vi "PH_PILS.set i attribute.vi"(0 "i ref in":refnum<vi>, 2 "i attribute":T1={"Boolean"=[], "GUI Refs Exp. Shutters"={"1"=refnum, "2"=refnum, "3"=refnum, "4"=refnum}, "Tristate2Run GUI Refs"=[], "EO-Likes"=[], "Operation Mode"={"Operation Mode"=enum."unknown", "GUI"={"Ref State"=refnum, "Ref"=refnum}, "Servicemode"={"Tagname"="", "Status"=0}, "Labormode"={"Tagname"="", "Status"=0}, "Searchmode"={"Tagname"="", "Status"=0}, "Shotmode"={"Tagname"="", "Status"=0}}, "Submode"={"Submode"=enum."unknown", "GUI"={"Ref State"=refnum, "Ref"=refnum}, "Submode"={"Tagname"="", "Status"=0}}, "Experiment"={"Experiment"=enum."unknown", "GUI"={"Ref State"=refnum, "Ref"=refnum}, "intern"={"Tagname"="", "Status"=0}, "Exp 4"={"Tagname"="", "Status"=0}, "Exp 3"={"Tagname"="", "Status"=0}, "Exp 2"={"Tagname"="", "Status"=0}, "Exp 1"={"Tagname"="", "Status"=0}}, "TristateNormal"=[], "Door Tags"=[], "GUIlessTags"=[], "Beamline GUI Refs"=[], "Special Boolean"=[], "Laserpower"=[], "Shutter"=[], "Tristate EO Like"=[], "PP"=[], "Switch Knobs"=[], "Latch Knob GUI Refs"=[], "FailureCounter"=0, "Enabled Status"={"Laser"=0, "PreAmp"=0, "MainAmp"=0}, "Mercury"=refnum, "Instance Rods"="N/A", "Logfile"=path "", "Beckhoff-Instance Internal"="", "Beckhoff-Instance External"="", "Enabling Rights"=[]}, 5 "error in (no error)":errorcluster) -> (14 "i ref out":refnum<vi>, 19 "error out":errorcluster)   [LabVIEW 2014, in "PH_PILS.lvlib"]
doc: "Sets the i attribute data of an object.\n\nLicense Agreement for this software:\n\nCopyright (C)\nGesellschaft für Schwerionenforschung, GSI\nPlanckstr. 1\n64291 Darmstadt\nGermany\n\nContact: D.Beck@gsi.de \n\nThis program is free software; you can redistribute it and/or modify it under the terms of the GNU General Public License as published by the Free Software Foundation; either version 2 of the license, or (at your option) any later version.\n\nThis program is distributed in the hope that it will be useful, but WITHOUT ANY WARRANTY; without even the implied warranty of MERCHANTABILITY or FITNESS FOR A PARTICULAR PURPOSE. See the GNU General License for more details (http://www.gnu.org).\n\nGesellschaft für Schwerionenforschung, GSI\nPlanckstr. 1, 64291 Darmstadt, Germany\nFor all questions and ideas contact: M.Richter@gsi.de, H.Brand@gsi.de or D.Beck@gsi.de.\nLast update: 17-JUN-2004"
uses:
  PH_PILS.lvlib
  PH_PILS.i attribute.ctl
  PH_PILS.Operation Mode.ctl
  PH_PILS.Submode.ctl
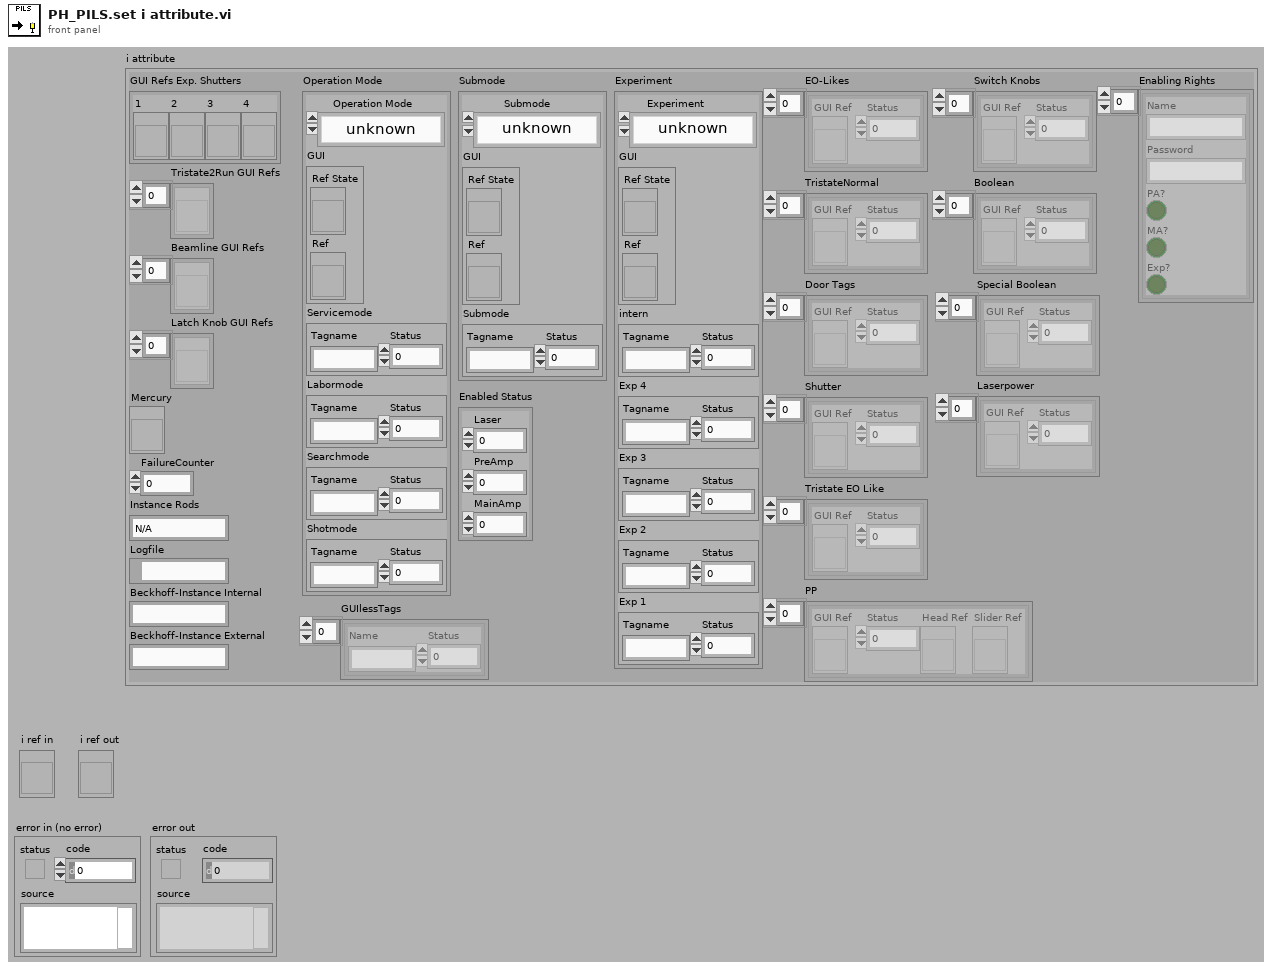
[diagram p1: front panel]
types:
  T1 = typedef "PH_PILS.lvlib/PH_PILS.i attribute.ctl" = cluster{"Boolean":cluster{"GUI Ref":refnum<vi>, "Status":i32}[], "GUI Refs Exp. Shutters":cluster{"1":refnum<vi>, "2":refnum<vi>, "3":refnum<vi>, "4":refnum<vi>}, "Tristate2Run GUI Refs":refnum<vi>[], "EO-Likes":cluster{"GUI Ref":refnum<vi>, "Status":i32}[], "Operation Mode":cluster{"Operation Mode":T2, "GUI":cluster{"Ref State":refnum<vi>, "Ref":refnum<vi>}, "Servicemode":cluster{"Tagname":string, "Status":i32}, "Labormode":cluster{"Tagname":string, "Status":i32}, "Searchmode":cluster{"Tagname":string, "Status":i32}, "Shotmode":cluster{"Tagname":string, "Status":i32}}, "Submode":cluster{"Submode":T3, "GUI":cluster{"Ref State":refnum<vi>, "Ref":refnum<vi>}, "Submode":cluster{"Tagname":string, "Status":i32}}, "Experiment":cluster{"Experiment":enum16{"unknown", "intern", "4 (Z6)", "3", "2", "1"}, "GUI":cluster{"Ref State":refnum<vi>, "Ref":refnum<vi>}, "intern":cluster{"Tagname":string, "Status":i32}, "Exp 4":cluster{"Tagname":string, "Status":i32}, "Exp 3":cluster{"Tagname":string, "Status":i32}, "Exp 2":cluster{"Tagname":string, "Status":i32}, "Exp 1":cluster{"Tagname":string, "Status":i32}}, "TristateNormal":cluster{"GUI Ref":refnum<vi>, "Status":i32}[], "Door Tags":cluster{"GUI Ref":refnum<vi>, "Status":i32}[], "GUIlessTags":cluster{"Name":string, "Status":i32}[], "Beamline GUI Refs":refnum<vi>[], "Special Boolean":cluster{"GUI Ref":refnum<vi>, "Status":i32}[], "Laserpower":cluster{"GUI Ref":refnum<vi>, "Status":i32}[], "Shutter":cluster{"GUI Ref":refnum<vi>, "Status":i32}[], "Tristate EO Like":cluster{"GUI Ref":refnum<vi>, "Status":i32}[], "PP":cluster{"GUI Ref":refnum<vi>, "Status":i32, "Head Ref":refnum<vi>, "Slider Ref":refnum<vi>}[], "Switch Knobs":cluster{"GUI Ref":refnum<vi>, "Status":i32}[], "Latch Knob GUI Refs":refnum<vi>[], "FailureCounter":i32, "Enabled Status":cluster{"Laser":i32, "PreAmp":i32, "MainAmp":i32}, "Mercury":refnum<vi>, "Instance Rods":string, "Logfile":path, "Beckhoff-Instance Internal":string, "Beckhoff-Instance External":string, "Enabling Rights":cluster{"Name":string, "Password":string, "PA?":bool, "MA?":bool, "Exp?":bool}[]}
  T2 = typedef "PH_PILS.lvlib/PH_PILS.Operation Mode.ctl" = enum16{"unknown", "Service", "Labor", "Search", "Shot"}
  T3 = typedef "PH_PILS.lvlib/PH_PILS.Submode.ctl" = enum16{"unknown", "HV-Normal", "HV-Test"}
  T4 = enum16{"SetAttribute", "GetAttribute", "CreateAttribute", "DestroyAttribute", "DestroyAllAtributes"}
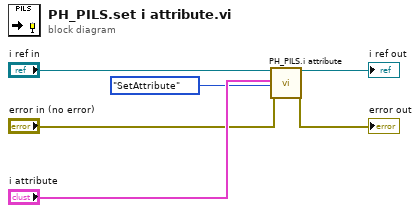
[diagram p0: block diagram]
diagram:
  n1 = call "PH_PILS.i attribute.vi"("VI Refnum"="i ref in", "CLASS.i attribute"="i attribute", "Action"=T4."SetAttribute", "error in (no error)"="error in (no error)") -> ("VI Refnum out"=→"i ref out":refnum<vi>, "error out"=→"error out":errorcluster)  [unwired: 13 in, 1 out]
